vi "Reader Listen.vi"(8 "error in (no error)":errorcluster, 11 "TCP Reader in":refnum<class "TCP Reader.lvclass">) -> (0 "error out":errorcluster, 3 "TCP Reader out":refnum<class "TCP Reader.lvclass">)   [LabVIEW 2012, in "TCP Classes.lvlib" / "TCP Reader.lvclass"]
uses:
  TCP Reader.lvclass
  Class TCP Connection/TCP Connection.lvclass/TCP Connection.ctl
  <userlib>/STM/TCP/stm_TCP Read Options.ctl
  <vilib>/ActorFramework/Actor/Actor.lvclass/Actor.ctl
  <vilib>/ActorFramework/Message Enqueuer/Message Enqueuer.lvclass/Message Enqueuer.ctl
  Class TCP Connection/Read Connection.vi
  <vilib>/ActorFramework/Message Enqueuer/Enqueue.vi
  <vilib>/ActorFramework/Message Enqueuer/Init from Existing Queue.vi
  Common/SubVIs/Conn Status Global.vi
  <userlib>/STM/TCP/STM Read Message (TCP).vi
  <vilib>/ActorFramework/Message Priority Queue/Priority Enqueue.vi
  Cfg Grandmaster/DAQMan Messages/Start DAQ Msg/Start DAQ Msg.lvclass
  Cfg Grandmaster/DAQMan Messages/Stop All DAQ Msg/Stop All DAQ Msg.lvclass
  <vilib>/ActorFramework/Message Enqueuer/Message Enqueuer.lvclass
  TCP Reader Messages/Listen Msg/Reader Listen Msg.lvclass
  Class TCP Connection/TCP Connection.lvclass
  <vilib>/ActorFramework/Actor/Actor.lvclass
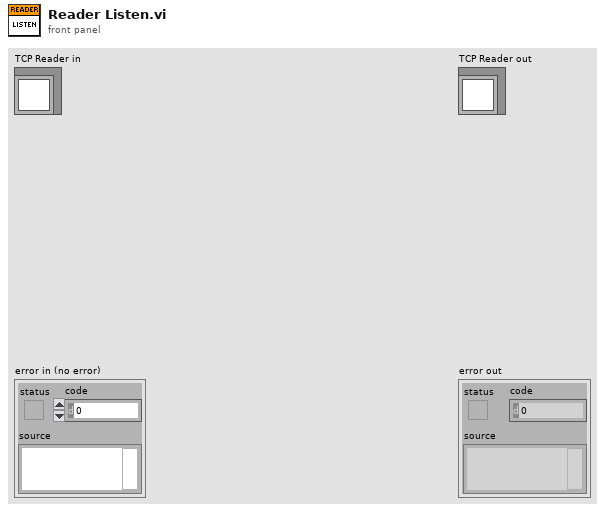
[diagram p1: front panel]
types:
  T1 = typedef "stm_TCP Read Options.ctl" = cluster{"Ignore Timeout Error":bool, "timeout ms (1000)":i32}
  T2 = typedef "stm_TCP Connection Info.ctl" = cluster{"connection ID":refnum<k5>, "Meta data":T3[]}
  T3 = typedef "stm_MetaDataElement.ctl" = string
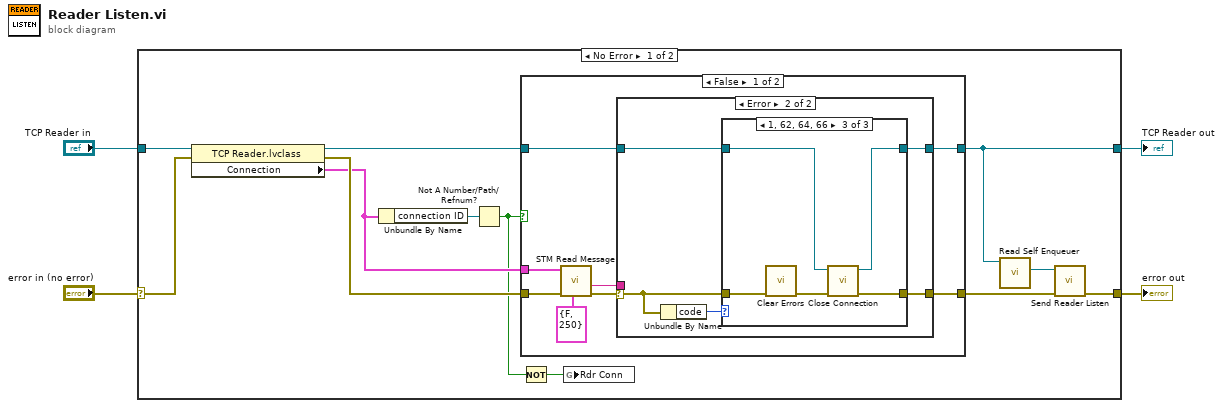
[diagram p0: block diagram]
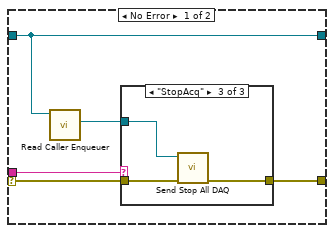
[diagram p2: hidden frame]
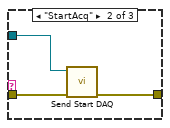
[diagram p4: hidden frame]
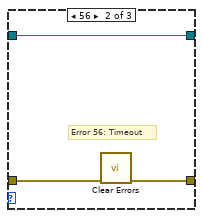
[diagram p6: hidden frame]
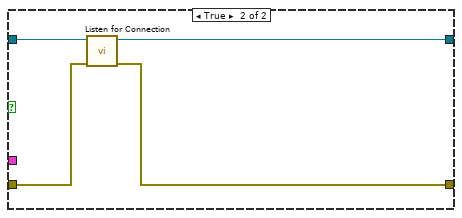
[diagram p7: hidden frame]
diagram:
  n1 = case shown="No Error" "error in (no error)" {
    selector: "error in (no error)" -> [w15 w57]
    tunnel: [w8 w57] -> w3
    tunnel: [w10 w56] -> w1
    tunnel: "TCP Reader in" -> [w16 w56]
    frame No Error {
      n2 = property class="TCP Reader.lvclass"(reference=w16, error in=w15) -> (reference out=w13:refnum<class "TCP Reader.lvclass">, error out=w12:errorcluster, "Connection"=w11:T2)
      n3 = Unbundle By Name(w11) -> ("connection ID"=w14:refnum<k5>)
      n4 = Not A Number/Path/Refnum?(number/path/refnum=w14) -> (NaN/Path/Refnum?=w5:bool)
      n5 = case shown="False" w5 {
        tunnel: w13 -> [w19 w55]
        tunnel: [w18 w54] -> w10
        tunnel: [w17 w52] -> w9
        tunnel: w12 -> [w23 w53]
        tunnel: w11 -> [w22 _]
        frame False {
          n6 = call-poly <userlib>:"STM Read Message.vi"("Options"=T1 {"Ignore Timeout Error"=FALSE, "timeout ms (1000)"=250}, "error in"=w23, "Connection Info"=w22) -> ("error out"=w21:errorcluster, "Name"=w20:T3)  [unwired: 3 in, 4 out]
          n7 = case shown="Error" w21 {
            selector: w21 -> [w28 w40]
            tunnel: [w27 w39] -> w17
            tunnel: w20 -> [w29 _]
            tunnel: w19 -> [w26 w38]
            tunnel: [w26 w37] -> w18
            frame No Error {
              n8 = call <vilib>:"Read Caller Enqueuer.vi"("Actor"=w26) -> ("Caller Enqueuer"=w25:refnum<class "Message Enqueuer.lvclass">)  [unwired: 10 in]
              n9 = case shown="\"StopAcq\"" w29 {
                tunnel: w28 -> [w30 w33 w35]
                tunnel: [w30 w32 w36] -> w27
                tunnel: w25 -> [_ w31 w34]
                frame Default {
                }
                frame "StartAcq" {
                  n10 = call "Send Start DAQ.vi"("error in (no error)"=w33, "Message Enqueuer"=w31) -> ("error out"=w32:errorcluster)  [unwired: 8 in, 1 out]
                }
                frame "StopAcq" {
                  n11 = call "Send Stop All DAQ.vi"("error in (no error)"=w35, "Message Enqueuer"=w34) -> ("error out"=w36:errorcluster)  [unwired: 8 in, 1 out]
                }
              }
            }
            frame Error {
              n12 = Unbundle By Name(w40) -> ("code"=w41:i32)
              n13 = case shown="1, 62, 64, 66" w41 {
                tunnel: [w43 w46 w47] -> w39
                tunnel: w40 -> [w43 w45 w51]
                tunnel: w38 -> [w42 w44 w49]
                tunnel: [w42 w44 w48] -> w37
                frame Default {
                }
                frame 56 {
                  # "Error 56: Timeout"
                  n14 = call <vilib>:"Clear Errors.vi"("error in (no error)"=w45) -> ("error out"=w46:errorcluster)  [unwired: 6 in]
                }
                frame 1, 62, 64, 66 {
                  n15 = call <vilib>:"Clear Errors.vi"("error in (no error)"=w51) -> ("error out"=w50:errorcluster)  [unwired: 6 in]
                  n16 = call "Close Connection.vi"("error in (no error)"=w50, "TCP Connection in"=w49) -> ("error out"=w47:errorcluster, "TCP Connection out"=w48:refnum<class "TCP Reader.lvclass">)  [unwired: 8 in]
                }
              }
            }
          }
        }
        frame True {
          n17 = call-dynamic "Listen for Connection.vi"("error in (no error)"=w53, "TCP Connection in"=w55) -> ("error out"=w52:errorcluster, "TCP Connection out"=w54:refnum<class "TCP Reader.lvclass">)  [unwired: 7 in, 1 out]
        }
      }
      n18 = Not(x=w5) -> (.not. x?=w6:bool)
      n19 = global write "Conn Status Global.vi" "Rdr Conn"(w6) -> ()
      n20 = call <vilib>:"Read Self Enqueuer.vi"("Actor"=w10) -> ("Self Enqueuer"=w7:refnum<class "Message Enqueuer.lvclass">)  [unwired: 10 in]
      n21 = call "Send Reader Listen.vi"("error in (no error)"=w9, "Message Enqueuer"=w7) -> ("error out"=w8:errorcluster)  [unwired: 8 in, 1 out]
    }
    frame Error {
    }
  }
  "error out" <- w3
  "TCP Reader out" <- w1
